vi "m1m3_getEvent_AccelerometerWarning.vi"(8 "error in (no error)":errorcluster, 11 "logevent_AccelerometerWarning_Ctl":T1) -> (0 "error out":errorcluster, 2 "function return":i32, 3 "logevent_AccelerometerWarning_Ctl out":T1)   [LabVIEW 2016, in "SALLV_m1m3.lvlib"]
doc: "int m1m3_shm_getEvent_AccelerometerWarningLV(m1m3_logevent_AccelerometerWarningLV *logevent_AccelerometerWarning_Ctl );"
uses:
  SALLV_m1m3.lvlib
  DataTypes/logevent_AccelerometerWarning.ctl
  SALLV_m1m3.so
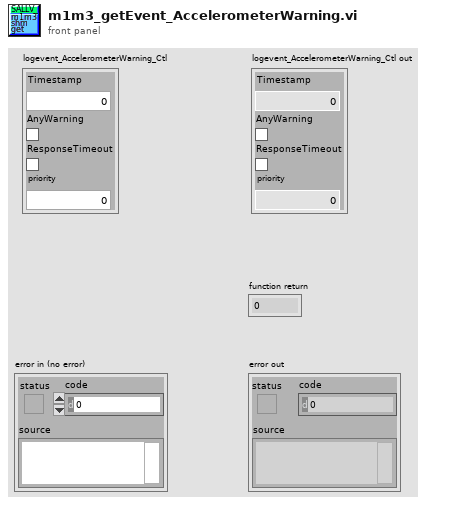
[diagram p1: front panel]
types:
  T1 = typedef "SALLV_m1m3.lvlib/logevent_AccelerometerWarning.ctl" = cluster{"Timestamp":dbl, "AnyWarning":bool, "ResponseTimeout":bool, "priority":i32}
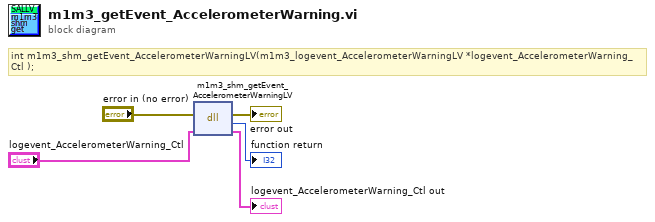
[diagram p0: block diagram]
diagram:
  # "int m1m3_shm_getEvent_AccelerometerWarningLV(m1m3_logevent_AccelerometerWarningLV *logevent_AccelerometerWarning_Ctl );"
  n1 = dll-call lib="opt/CODE/SALLV_m1m3/SALLV_m1m3.*" fn="m1m3_shm_getEvent_AccelerometerWarningLV"(error in="error in (no error)", "logevent_AccelerometerWarning_Ctl"="logevent_AccelerometerWarning_Ctl") -> (error out=→"error out":errorcluster, →"function return":i32, "logevent_AccelerometerWarning_Ctl"=→"logevent_AccelerometerWarning_Ctl out":T1)  [unwired: 2 in, 1 out]
